vi "Create Virtual Folder.vi"(8 "error in (no error)":errorcluster, 10 "Folder Config":T1, 11 "Library":refnum<vi>) -> (0 "error out":errorcluster, 3 "Folder Ref":refnum<vi>)   [LabVIEW 2020, in "Negentropic IDE.lvlib"]
uses:
  Negentropic IDE.lvlib
  Folder Config.ctl
  Scope.ctl
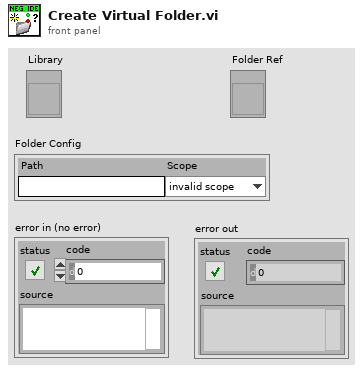
[diagram p1: front panel]
types:
  T1 = typedef "Negentropic IDE.lvlib/Folder Config.ctl" = cluster{"Path":string, "Scope":T2}
  T2 = typedef "Negentropic IDE.lvlib/Scope.ctl" = enum32{"invalid scope", "public", "private", "protected", "community"}
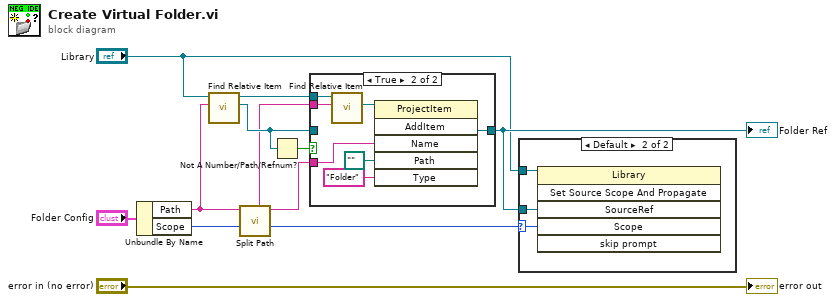
[diagram p0: block diagram]
diagram:
  n1 = Unbundle By Name("Folder Config") -> ("Path"=w6:string, "Scope"=w10:T2)
  n2 = call "Find Relative Item.vi"("Item Path"=w6, "Root Item In"="Library") -> ("Item Ref"=w4:refnum<vi>, "Root Item"=w2:refnum<vi>)  [unwired: 7 in, 1 out]
  n3 = call "Split Path.vi"("Item Path"=w6) -> ("Item Name"=w8:string, "Parent Path"=w3:string)  [unwired: 9 in]
  n4 = Not A Number/Path/Refnum?(number/path/refnum=w4) -> (NaN/Path/Refnum?=w5:bool)
  n5 = case shown="True" w5 {
    tunnel: w8 -> [_ w19]
    tunnel: [w12 w18] -> w9
    tunnel: w4 -> [w12 _]
    tunnel: w3 -> [_ w15]
    tunnel: w2 -> [_ w14]
    frame False {
    }
    frame True {
      n6 = call "Find Relative Item.vi"("Item Path"=w15, "Root Item In"=w14) -> ("Item Ref"=w13:refnum<vi>)  [unwired: 7 in, 2 out]
      n7 = invoke class="ProjectItem" method="AddItem"(reference=w13, "Name"=w19, "Path"=path "", "Type"="Folder") -> ("AddItem"=w18:refnum<vi>)  [unwired: 2 in, 5 out]
    }
  }
  "Folder Ref" <- w9
  n8 = case shown="Default" w10 {
    selector: w10 -> [_ w21]
    tunnel: "Library" -> [_ w22]
    tunnel: w9 -> [_ w20]
    frame "invalid scope" {
    }
    frame Default {
      n9 = invoke class="Library" method="Set Source Scope And Propagate"(reference=w22, "SourceRef"=w20, "Scope"=w21) -> ()  [unwired: 3 in, 6 out]
    }
  }
  "error out" <- "error in (no error)"
